vi "Apply View to Tree Control.vi"(7 "View Mode":T2, 8 "error in (no error)":errorcluster, 10 "refnum":T1, 11 "TreeControl in":refnum<vi>) -> (0 "error out":errorcluster)   [LabVIEW 2017]
uses:
  View Mode.ctl
  DSF Configuration API/1.0.0/Public/Controls/DSF Config Data RefNum.ctl
  DSF Configuration API/1.0.0/DSF Configuration API.lvlib
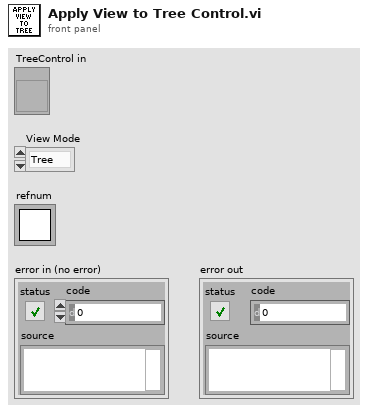
[diagram p1: front panel]
types:
  T1 = typedef "DSF Configuration API.lvlib/DSF Config Data RefNum.ctl" = refnum<k1>
  T2 = typedef "View Mode.ctl" = enum16{"Tree", "List"}
  T3 = cluster{"Left Cell String":string, "Child Text":string[], "Child Tag":string, "Item Indent":i32, "Child Only?":bool, "Glyph Index":i32}[]
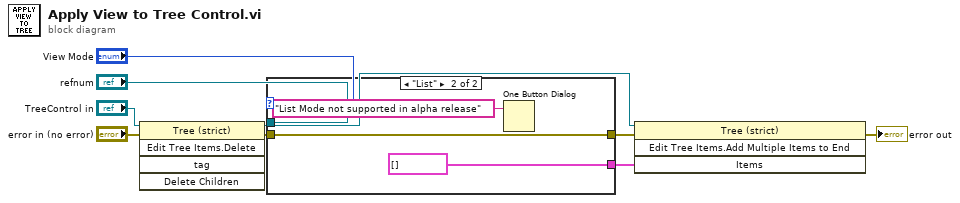
[diagram p0: block diagram]
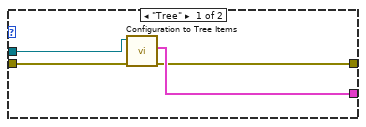
[diagram p2: hidden frame]
diagram:
  n1 = invoke class="Tree (strict)" method="Edit Tree Items.Delete"(reference="TreeControl in", error in="error in (no error)") -> (reference out=w2:refnum<vi>, error out=w8:errorcluster)  [unwired: 3 in, 3 out]
  n2 = case shown="\"List\"" "View Mode" {
    tunnel: "refnum" -> [w13 _]
    tunnel: [w12 T3 [] ("Items")] -> w4
    tunnel: w8 -> [w11 w15]
    tunnel: [w10 w15] -> w9
    frame "Tree" {
      n3 = call "Configuration to Tree Items.vi"("error in (no error)"=w11, "Refnum In"=w13) -> ("error out"=w10:errorcluster, "Items"=w12:T3)  [unwired: 7 in, 1 out]
    }
    frame "List" {
      n4 = One Button Dialog(message="List Mode not supported in alpha release") -> ()  [unwired: 1 in, 1 out]
    }
  }
  n5 = invoke class="Tree (strict)" method="Edit Tree Items.Add Multiple Items to End"(reference=w2, error in=w9, "Items"=w4) -> (error out=→"error out":errorcluster)  [unwired: 1 in, 3 out]
